vi "holoTrackPath.vi"() -> (3 "appended path":path)   [LabVIEW 2023, in "holoPyTracks.lvlib"]
uses:
  holoPyTracks.lvlib
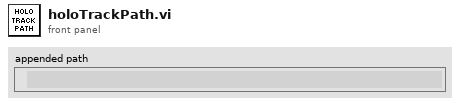
[diagram p1: front panel]
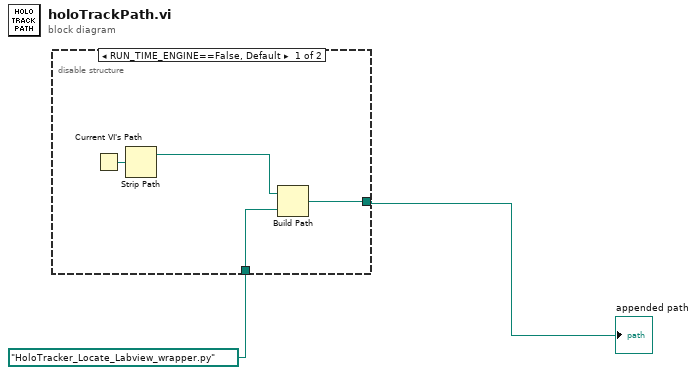
[diagram p0: block diagram]
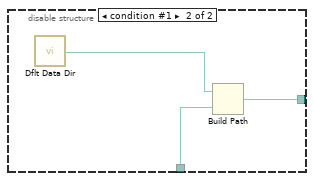
[diagram p2: hidden frame]
diagram:
  n1 = disable-structure shown="RUN_TIME_ENGINE==False, Default" {
    disable-tunnel: [w4 w9] -> w2
    disable-tunnel: path "HoloTracker_Locate_Labview_wrapper.py" ("name or relative path") -> [w3 w7]
    frame condition #0 (active) {
      n2 = Current VI's Path() -> (path=w5:path)
      n3 = Strip Path(path=w5) -> (stripped path=w6:path)  [unwired: 1 out]
      n4 = Build Path(base path=w6, name or relative path=w3) -> (appended path=w4:path)
    }
    frame condition #1 {
      n5 = call <vilib>:"Dflt Data Dir.vi"() -> ("App:Default Data Directory"=w8:path)
      n6 = Build Path(base path=w8, name or relative path=w7) -> (appended path=w9:path)
    }
  }
  "appended path" <- w2
